vi "Shooter - Calculate Hood Angle (SubVI).vi"(6 "shooterVelocityDesired In":dbl, 7 "v slope":dbl=0.35, 9 "distance in":dbl, 10 "x slope":dbl=-1.5, 11 "71. hoodRegressionYInt":dbl) -> (1 "v*slope multiple":dbl, 2 "hood counts":dbl, 3 "x*slope multiple":dbl)   [LabVIEW 2019]
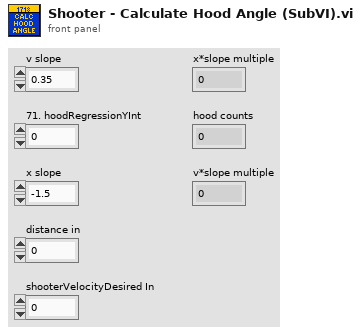
[diagram p1: front panel]
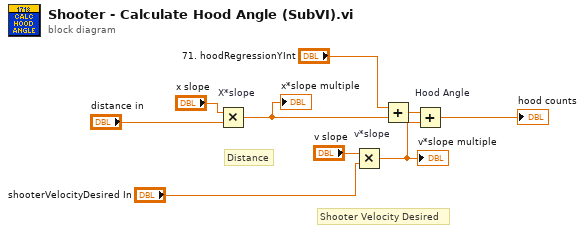
[diagram p0: block diagram]
diagram:
  # "Shooter Velocity Desired"
  # "Distance"
  n1 = Multiply "X*slope"(x="x slope", y="distance in") -> (x*y=w3:dbl)
  "x*slope multiple" <- w3
  n2 = Multiply "v*slope"(x="v slope", y="shooterVelocityDesired In") -> (x*y=w2:dbl)
  "v*slope multiple" <- w2
  n3 = Add ("Add Intercept")(x="71. hoodRegressionYInt", y=w3) -> (x+y=w1:dbl)
  n4 = Add "Hood Angle"(x=w1, y=w2) -> (x+y=→"hood counts":dbl)
